vi "ShooterWrapper.vi"(6 "Action":T1, 7 "error in":errorcluster, 10 "ShooterWait":i32=750) -> (0 "error out":errorcluster)   [LabVIEW 2013]
doc: "CheckedShooter is used during a normal shooting sequence (either during one-ball autonomous or teleop). It controls the shooting pneumatics (through Shooter.vi), but it ALSO checks preconditions: the collector arm, the clappers, and the roller. It has the following actions:\n-Init: take two double solenoid references and store them (one for the clapper, one for the roller). Take two single solenoid references and use them to initialize Shooter.vi (one for the firing cylinder, one for the kicker).\n-Shoot:\n +Check if the collector is up (hitting the top limit switch). (Only if CheckLimitSwitch is true.)\n +Actuate the roller to out.\n +Actuate the clapper to middle.\n +Shoot (using Shooter.vi). Wait1, Wait2, and Wait3 correspond to the waits used by Shooter.vi."
uses:
  ShooterWrapperAction.ctl
  LEDSaction.ctl
  ShooterAction.ctl
  DoubleSolenoidAction.ctl
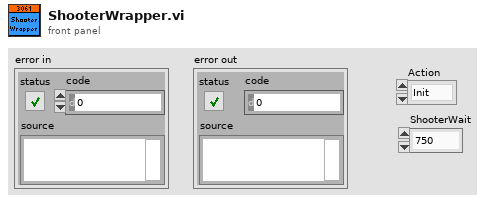
[diagram p1: front panel]
types:
  T1 = typedef "ShooterWrapperAction.ctl" = enum16{"Init", "CollectorDown", "CollectorUp"}
  T2 = typedef "LEDSaction.ctl" = enum16{"Init", "10SecondsLeft", "LimitDown", "LimitUp", "CollectDown", "CollectUp", "NotHot", "Hot", "Shift", "RollBack", "RollFwd", "Shoot", "Distance Low", "DistanceHigh", "PressureLow", "PressureHigh"}
  T3 = typedef "ShooterAction.ctl" = enum16{"Init", "Shoot"}
  T4 = typedef "DoubleSolenoidAction.ctl" = enum16{"Init", "Middle", "In", "Out"}
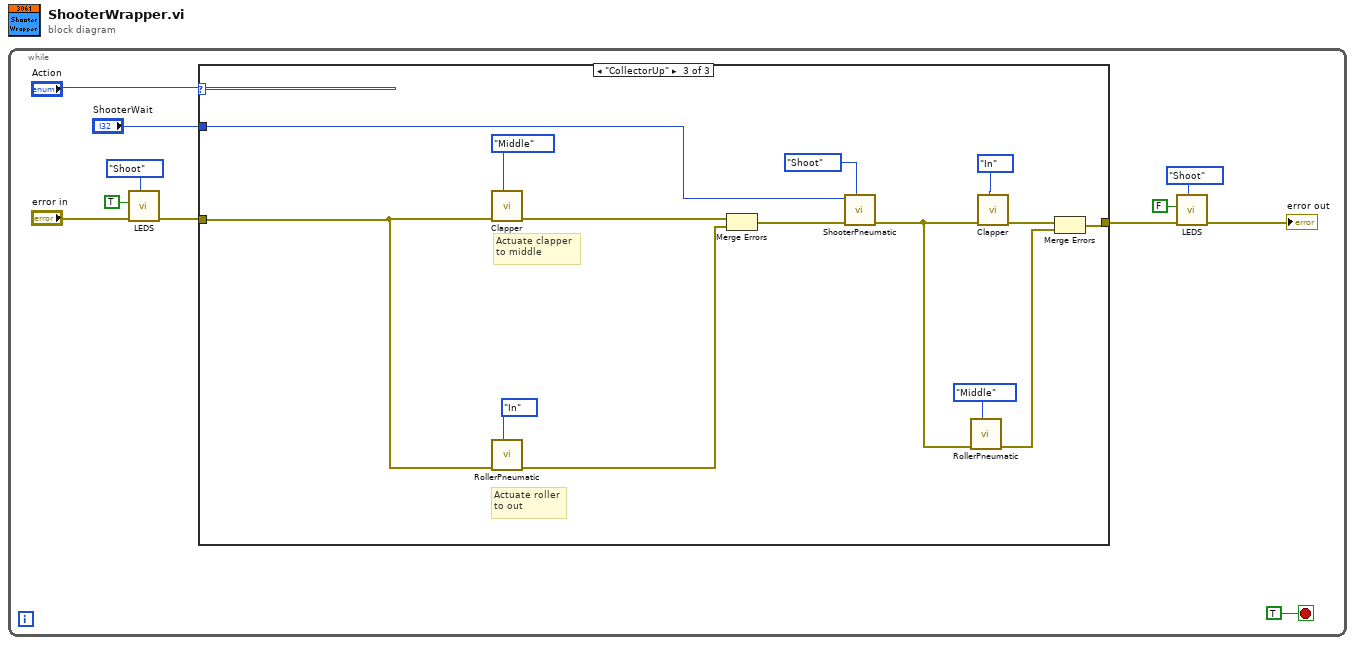
[diagram p0: block diagram]
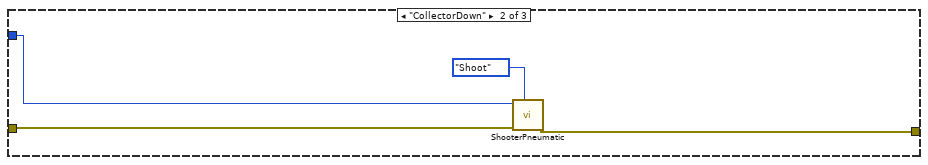
[diagram p3: hidden frame]
diagram:
  n1 = while {
    stop <- TRUE stop-if-true
    n2 = call "LEDS.vi"("Action"=LEDSaction."Shoot", "error in"="error in", "On/Off"=TRUE) -> ("error out"=w7:errorcluster)  [unwired: 8 in]
    n3 = case shown="\"CollectorUp\"" "Action" {
      tunnel: w7 -> [w12 w14 w24]
      tunnel: [w12 w15 w20] -> w8
      tunnel: "ShooterWait" -> [_ w13 w17]
      frame "Init", Default {
      }
      frame "CollectorDown" {
        n4 = call "ShooterPneumatic.vi"("Action"=ShooterAction."Shoot", "error in"=w14, "Wait1"=w13) -> ("error out"=w15:errorcluster)  [unwired: 8 in]
      }
      frame "CollectorUp" {
        # "Actuate clapper\nto middle"
        # "Actuate roller\nto out"
        n5 = call "Clapper.vi"("State"=DoubleSolenoidAction."Middle", "Error in"=w24) -> ("Error out"=w26:errorcluster)  [unwired: 9 in]
        n6 = call "RollerPneumatic.vi"("State"=DoubleSolenoidAction."In", "Error in"=w24) -> ("Error out"=w25:errorcluster)  [unwired: 9 in]
        n7 = Merge Errors(w26, w25) -> (w27:errorcluster)
        n8 = call "ShooterPneumatic.vi"("Action"=ShooterAction."Shoot", "error in"=w27, "Wait1"=w17) -> ("error out"=w21:errorcluster)  [unwired: 8 in]
        n9 = call "RollerPneumatic.vi"("State"=DoubleSolenoidAction."Middle", "Error in"=w21) -> ("Error out"=w18:errorcluster)  [unwired: 9 in]
        n10 = call "Clapper.vi"("State"=DoubleSolenoidAction."In", "Error in"=w21) -> ("Error out"=w19:errorcluster)  [unwired: 9 in]
        n11 = Merge Errors(w19, w18) -> (w20:errorcluster)
      }
    }
    n12 = call "LEDS.vi"("Action"=LEDSaction."Shoot", "error in"=w8, "On/Off"=FALSE) -> ("error out"=→"error out":errorcluster)  [unwired: 8 in]
  }
